vi "Test Find Dashed Tests.vi"(8 "error in (no error)":errorcluster, 11 "Test Case In":refnum<class "Test FInder Test.lvclass">) -> (0 "error out":errorcluster, 3 "Test Case Out":refnum<class "Test FInder Test.lvclass">)   [LabVIEW 2020, in "Test FInder Test.lvclass"]
uses:
  Test FInder Test.lvclass
  Test FInder Test.lvclass/Test FInder Test.ctl
  source/Framework/Test Finder/Test Finder.lvclass
  <vilib>/Astemes/LUnit/Test Case.lvclass
  source/LUnit Test Suite.lvclass
  C:/git/astemes-lunit/source/Core/Runnable/Runnable.lvclass
  C:/Program Files (x86)/National Instruments/LabVIEW 2020/vi.lib/Astemes/LUnit/Test Case.lvclass
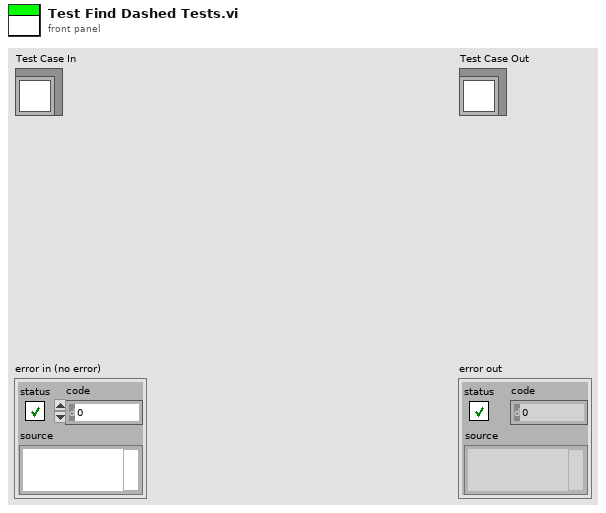
[diagram p1: front panel]
types:
  T1 = typedef "Result.lvlib/Result.ctl" = cluster{"Name":string, "Description":string, "Status":T2, "Result Type":T3, "Execution Time":dbl, "Data":cluster{"Expected":variant, "Actual":variant, "Delta":variant}}
  T2 = typedef "Result.lvlib/Status.ctl" = enum16{"", "Passed", "Failed", "Error", "Skipped", "Setup Error", "Broken", "Teardown Error"}
  T3 = typedef "Result.lvlib/Type.ctl" = enum16{"Test Case", "Test Suite", "Test Run", "Pass", "Fail", "Skip", "Pass if", "Fail if", "Pass if Error", "Fail if Error", "Pass if Equal", "Fail if Equal"}
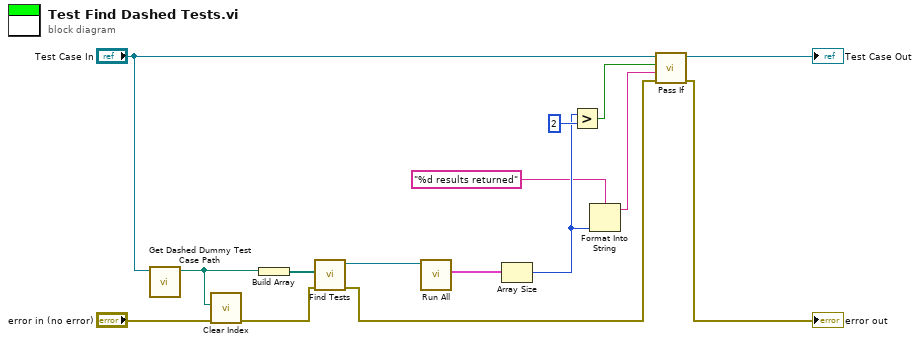
[diagram p0: block diagram]
diagram:
  n1 = call "Get Dashed Dummy Test Case Path.vi"("LUnit Test Suite Tests in"="Test Case In") -> ("appended path"=w1:path)  [unwired: 10 in]
  n2 = call "Clear Index.vi"("error in (no error)"="error in (no error)", "Project Path"=w1) -> ("error out"=w2:errorcluster)  [unwired: 9 in]
  n3 = Build Array(w1) -> (w12:path[])
  n4 = call "Find Tests.vi"("error in (no error)"=w2, "File Paths"=w12) -> ("error out"=w13:errorcluster, "LUnit Test Suite"=w11:refnum<class "LUnit Test Suite.lvclass">)  [unwired: 8 in]
  n5 = call "Run All.vi"("Runnable In"=w11) -> ("Results"=w10:T1[])  [unwired: 9 in, 1 out]
  n6 = Array Size(array=w10) -> (size(s)=w5:i32)
  n7 = Greater?(x=w5, y=2) -> (0:w6:bool)
  n8 = Format Into String(format string="%d results returned", w5) -> (resulting string=w3:string)  [unwired: 2 in, 1 out]
  n9 = call <vilib>:"Pass If.vi"("error in (no error)"=w13, "Message"=w3, "Pass?"=w6, "LUnit Test Case In"="Test Case In") -> ("error out"=→"error out":errorcluster, "LUnit Test Case Out"=→"Test Case Out":refnum<class "Test FInder Test.lvclass">)  [unwired: 6 in]
